vi "arduino sensirion serial setup (sub-vi).vi"(8 "error in (no error)":errorcluster, 10 "baud rate (576000)":u32=576000) -> (0 "error out":errorcluster, 3 "VISA resource name out":refnum<visa-resource-name>)   [LabVIEW 2021]
uses:
  <vilib>/Instr/_visa.llb/VISA Configure Serial Port (Instr).vi
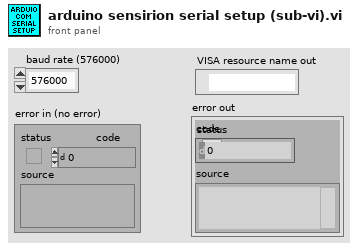
[diagram p1: front panel]
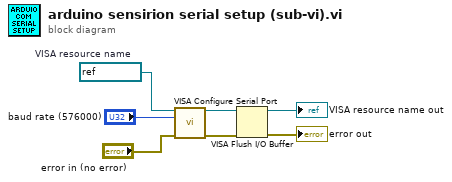
[diagram p0: block diagram]
diagram:
  w6 = refnum<visa-resource-name> "COM3"  # VISA resource name
  n1 = call-poly "VISA Configure Serial Port"("VISA resource name"=w6, "baud rate (9600)"="baud rate (576000)", "error in (no error)"="error in (no error)") -> ("VISA resource name out"=w5:refnum<visa-resource-name>, "error out"=w4:errorcluster)  [unwired: 11 in]
  n2 = VISA Flush I/O Buffer(VISA resource name=w5, error in (no error)=w4) -> (VISA resource name out=→"VISA resource name out":refnum<visa-resource-name>, error out=→"error out":errorcluster)  [unwired: 1 in]
